vi "Trial Timestamp Into DB.vi"(8 "error in (no error)":errorcluster, 11 "MatlabExperiment in":refnum<class "MatlabExperiment.lvclass">) -> (0 "error out":errorcluster, 3 "MatlabExperiment out":refnum<class "MatlabExperiment.lvclass">)   [LabVIEW 2011, in "MatlabExperiment.lvclass"]
uses:
  MatlabExperiment.lvclass
  Acquisition/Database/StimulationPrimary.ctl
  <vilib>/addons/database/NI_Database_API.lvlib
  Acquisition/AcquistionObject/AcquistionObject.lvclass
panel:
  in  "time":timestamp
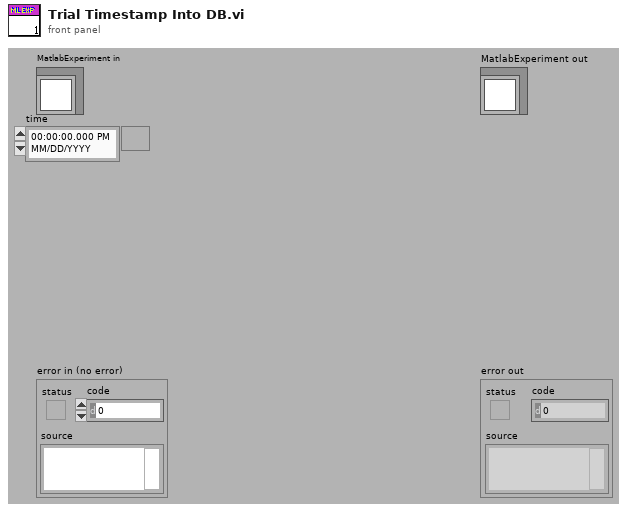
[diagram p1: front panel]
types:
  T1 = cluster{"setup":u8, "session_start_time":u64, "stim_start_time":u64, "time":u64}
  T2 = typedef "NI_Database_API.lvlib/Conn ObjectReference.ctl" = refnum<k1>
  T3 = typedef "StimulationPrimary.ctl" = cluster{"setup":u8, "subject_id":i32, "session_start_time":dbl, "stim_start_time":dbl}
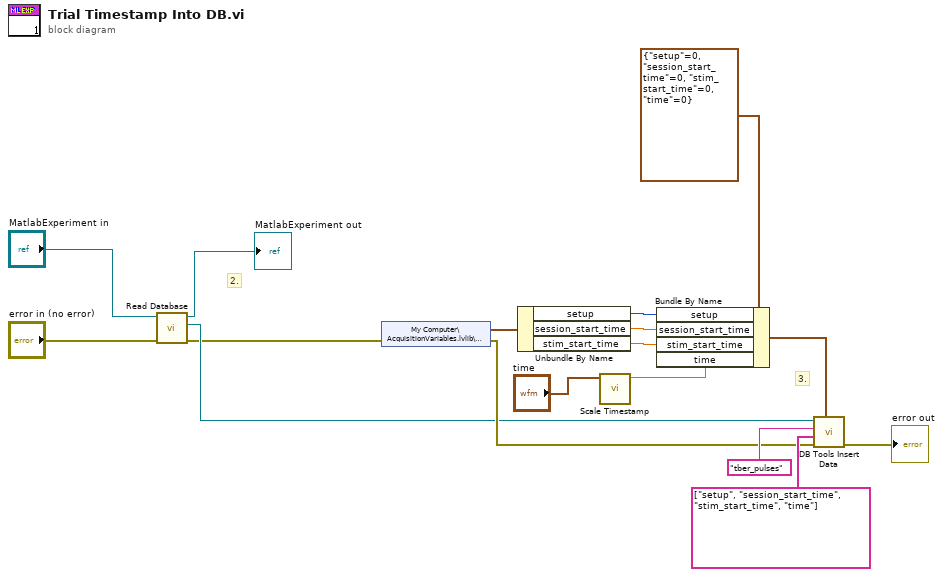
[diagram p0: block diagram]
diagram:
  # "2."
  # "3."
  n1 = call-dynamic "Read Database.vi"("error in (no error)"="error in (no error)", "AcquistionObject in"="MatlabExperiment in") -> ("error out"=w8:errorcluster, "reference"=w10:T2, "AcquistionObject out"=→"MatlabExperiment out":refnum<class "MatlabExperiment.lvclass">)  [unwired: 7 in]
  n2 = shared-variable "My Computer\\AcquisitionVariables.lvlib\\StimulationPK"(error in=w8) -> (w12:T3, error out=w11:errorcluster)
  n3 = Unbundle By Name(w12) -> ("setup"=w15:u8, "session_start_time"=w14:dbl, "stim_start_time"=w6:dbl)
  n4 = call "Scale Timestamp.vi"("Time Stamp"="time") -> ("Scaled timestamp"=w1:dbl)  [unwired: 10 in]
  n5 = Bundle By Name(cluster=T1 {"setup"=0, "session_start_time"=0, "stim_start_time"=0, "time"=0} ("Cluster"), "setup"=w15, "session_start_time"=w14, "stim_start_time"=w6, "time"=w1) -> (w13:T1)
  n6 = call <vilib>:"DB Tools Insert Data.vi"("data"=w13, "error in (no error)"=w11, "columns"=string[] ["setup", "session_start_time", "stim_start_time", "time"], "table"="tber_pulses", "connection reference"=w10) -> ("error out"=→"error out":errorcluster)  [unwired: 5 in, 1 out]
